vi "filters.vi"() -> ()   [LabVIEW 2025]
panel:
  out "bandpass":dynamicdata(graph)
  out "LOW PASS SIGNAL":dynamicdata(graph)
  out "concatination of two signals":dynamicdata(graph)
  out "HIGH PASS":dynamicdata(graph)
  out "SINE2":dynamicdata(graph)
  out "sine waveform":dynamicdata(graph)
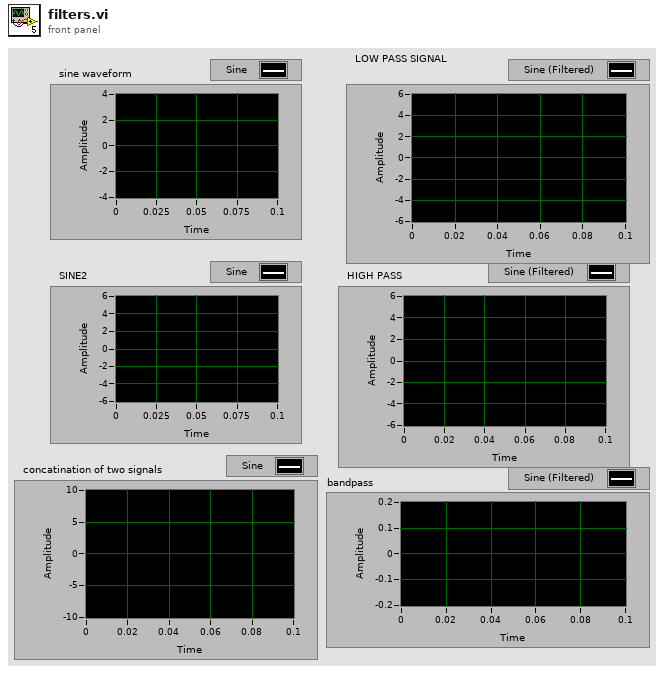
[diagram p1: front panel]
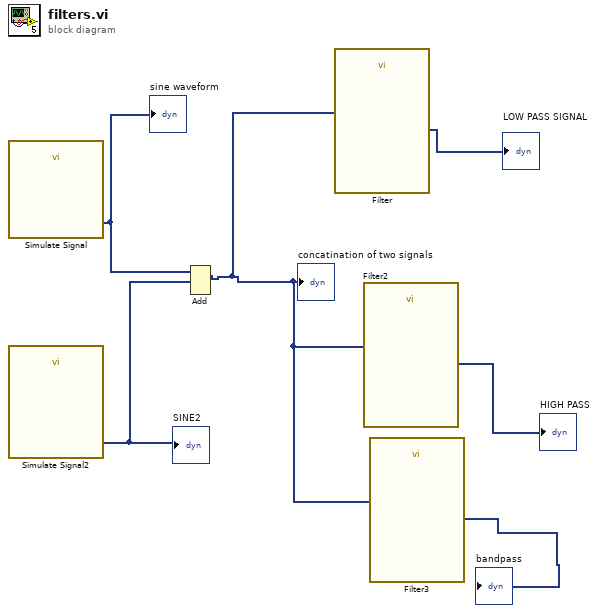
[diagram p0: block diagram]
diagram:
  n1 = call "Simulate Signal"() -> ("Sine"=w3:dynamicdata)  [unwired: 14 in, 1 out]
  "sine waveform" <- w3
  n2 = call "Simulate Signal2"() -> ("Sine"=w6:dynamicdata)  [unwired: 14 in, 1 out]
  "SINE2" <- w6
  n3 = Add(1:w6, 2:w3) -> (0:w2:dynamicdata)  [unwired: 1 in, 1 out]
  "concatination of two signals" <- w2
  n4 = call "Filter"("Signal"=w2) -> ("Filtered Signal"=→"LOW PASS SIGNAL":dynamicdata)  [unwired: 9 in, 1 out]
  n5 = call "Filter2"("Signal"=w2) -> ("Filtered Signal"=→"HIGH PASS":dynamicdata)  [unwired: 9 in, 1 out]
  n6 = call "Filter3"("Signal"=w2) -> ("Filtered Signal"=→"bandpass":dynamicdata)  [unwired: 9 in, 1 out]
